vi "Get Sensor Size.vi"(8 "error in (no error)":errorcluster, 11 "Camera in":refnum<class "Camera.lvclass">) -> (0 "error out":errorcluster, 2 "Sensor Size":T1, 3 "Camera":refnum<class "Camera.lvclass">)   [LabVIEW 2020, in "Camera.lvclass"]
uses:
  Camera.lvclass
  Buffer/Image Size.ctl
  Camera.lvclass/Camera.ctl
  Buffer/Buffer.lvclass
  bin/gindustrialcam_32-1.dll
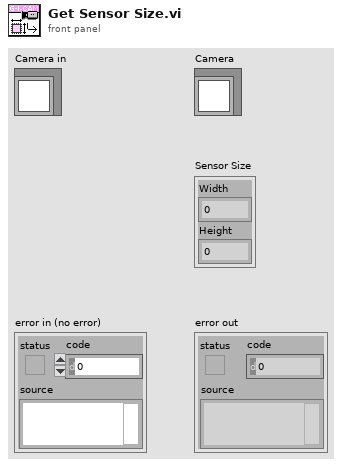
[diagram p1: front panel]
types:
  T1 = typedef "Buffer.lvclass/Image Size.ctl" = cluster{"Width":u16, "Height":u16}
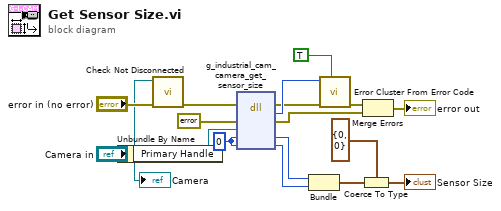
[diagram p0: block diagram]
diagram:
  w1 = 0 ("width")
  n1 = Unbundle By Name("Camera in") -> ("Primary Handle"=w12:refnum<data-value>)
  n2 = call "Check Not Disconnected.vi"("error in (no error)"="error in (no error)", "Camera in"="Camera in") -> ("error out"=w11:errorcluster)  [unwired: 9 in]
  n3 = dll-call lib="C:/serenial/lib/g-industrial-camera/LabVIEW/g_industrial_cam/bin/gindustrialcam_*-1.*" fn="g_industrial_cam_camera_get_sensor_size"(error in=w11, "err"=errorcluster {"status"=FALSE, "code"=0, "source"=""} ("error constant"), "edvr"=w12, "width"=w1, "height"=w1) -> (error out=w6:errorcluster, "Mg_Error"=w7:i32, "err"=w9:errorcluster, "width"=w5:i32, "height"=w4:i32)  [unwired: 3 in, 1 out]
  n4 = Bundle("width"=w5, "height"=w4) -> (w14:cluster{"width":i32, "height":i32})  [unwired: 1 in]
  n5 = call <vilib>:"Error Cluster From Error Code.vi"("show call chain? (False)"=TRUE, "error in (no error)"=w6, "error code (0)"=w7) -> ("error out"=w8:errorcluster)  [unwired: 6 in]
  n6 = Coerce To Type(0:w14, 1:T1 {"Width"=0, "Height"=0} ("Image Size")) -> (2:→"Sensor Size":T1)
  n7 = Merge Errors(w8, w9) -> (→"error out":errorcluster)
  "Camera" <- "Camera in"
